vi "Proportional Control.vi"(0 "Target Value X":dbl, 5 "Tolerance":dbl, 7 "Gain G":dbl, 9 "Current Value X":dbl, 13 "y OLD":dbl) -> (2 "y NEW":dbl, 6 "Adjustment":T1={"up"=FALSE, "down"=TRUE}, 8 "SHP Target Met":bool=TRUE)   [LabVIEW 2020]
uses:
  LabVIEW TOOLBOX VIs/Adjustment.ctl
panel:
  in  "Default Adjustment":T1={"up"=FALSE, "down"=TRUE}
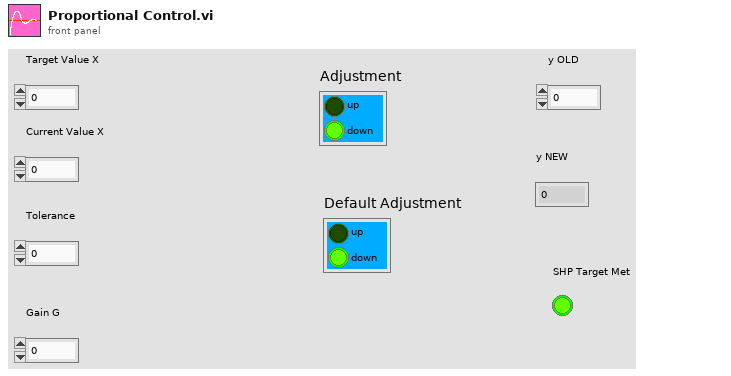
[diagram p1: front panel]
types:
  T1 = typedef "Adjustment.ctl" = cluster{"up":bool, "down":bool}
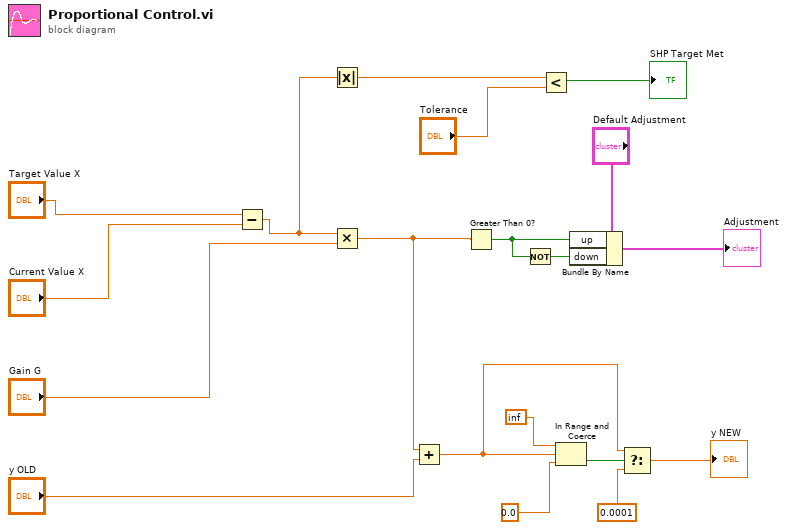
[diagram p0: block diagram]
diagram:
  n1 = Subtract(x="Target Value X", y="Current Value X") -> (x-y=w16:dbl)
  n2 = Absolute Value(x=w16) -> (abs(x)=w14:dbl)
  n3 = Multiply(x=w16, y="Gain G") -> (x*y=w15:dbl)
  n4 = Add(x=w15, y="y OLD") -> (x+y=w8:dbl)
  n5 = Greater Than 0?(x=w15) -> (x > 0?=w4:bool)
  n6 = Not(x=w4) -> (.not. x?=w5:bool)
  n7 = Less?(x=w14, y="Tolerance") -> (x < y?=→"SHP Target Met":bool)
  n8 = In Range and Coerce(upper limit=inf, x=w8, lower limit=0.0) -> (In Range?=w9:bool)  [unwired: 1 out]
  n9 = Bundle By Name(cluster="Default Adjustment", "up"=w4, "down"=w5) -> (→"Adjustment":T1)
  n10 = Select(t=w8, s=w9, f=0.0001) -> (s? t:f=→"y NEW":dbl)
